vi "FdxCmdTMGetRequestNumberCvi.vi"(8 "error in":errorcluster, 10 "TMHandle":u32, 11 "InstrumentHandle":u32) -> (0 "error out":errorcluster, 1 "RequestNumber":u16, 2 "TMHandleOut":u32, 3 "InstrumentHandle":u32)   [LabVIEW 2020, in "AIM664LV.lvlib"]
doc: "This function is used to get the request number for the next Time Manager Iteration."
uses:
  AIM664LV.lvlib
  AFDX_LibraryAdmin/FdxGlobalDllPath.vi
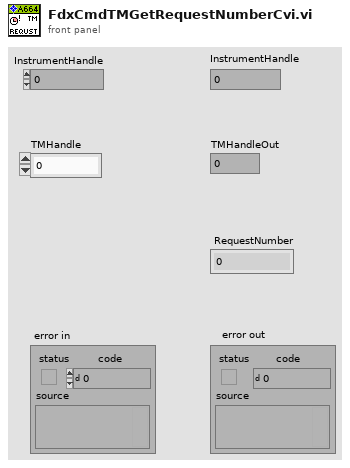
[diagram p1: front panel]
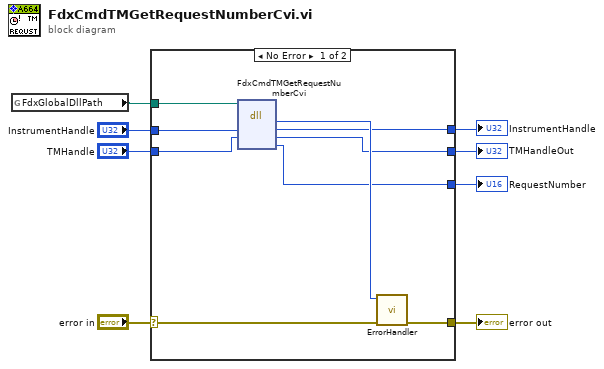
[diagram p0: block diagram]
diagram:
  n1 = global read "FdxGlobalDllPath.vi" "FdxGlobalDllPath"() -> (w6:path)
  n2 = case shown="No Error" "error in" {
    selector: "error in" -> [w16 w20]
    tunnel: [w17 w20] -> w8
    tunnel: w6 -> [w14 _]
    tunnel: "InstrumentHandle" -> [w13 w19]
    tunnel: [w12 w19] -> w4
    tunnel: "TMHandle" -> [w11 w18]
    tunnel: [w10 _] -> w2
    tunnel: [w9 w18] -> w1
    frame No Error {
      n3 = dll-call lib="aim_fdx.19.dll" fn="FdxCmdTMGetRequestNumberCvi" label="FdxCmdTMGetReuestNumber"(path in=w14, "InstrumentHandle"=w13, "TMHandle"=w11) -> ("status"=w15:i32, "InstrumentHandle"=w12:u32, "TMHandle"=w9:u32, "RequestNumber"=w10:u16)  [unwired: 2 in, 3 out]
      n4 = call "ErrorHandler.vi"("error in"=w16, "AIM Error"=w15) -> ("error out"=w17:errorcluster)  [unwired: 9 in]
    }
    frame Error {
    }
  }
  "error out" <- w8
  "InstrumentHandle" <- w4
  "RequestNumber" <- w2
  "TMHandleOut" <- w1
